vi "testSavedWithIdleTimeoutVisible.vi"(8 "error in (no error)":errorcluster, 11 "testStateMachineUtilities in":refnum<class "testStateMachineUtilities.lvclass">) -> (0 "error out":errorcluster, 3 "testStateMachineUtilities out":refnum<class "testStateMachineUtilities.lvclass">)   [LabVIEW 2013, in "testStateMachineUtilities.lvclass"]
uses:
  testStateMachineUtilities.lvclass
  <vilib>/Utility/traverseref.llb/TRef TravTarget.ctl
  <vilib>/Utility/traverseref.llb/VI Scripting - Traverse.lvlib
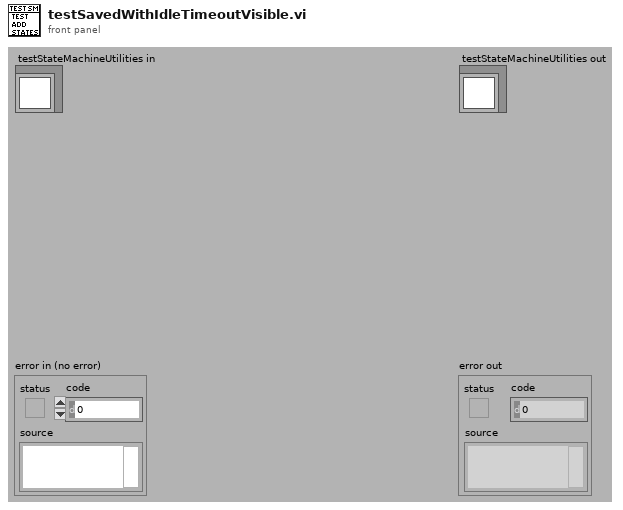
[diagram p1: front panel]
types:
  T1 = enum32{"Invalid", "Standard", "Closed", "Hidden", "Minimized", "Maximized"}
  T2 = typedef "TRef TravTarget.ctl" = enum16{"FP", "BD", "Other"}
  T3 = cluster{i32, refnum<vi>, "FrameNames":string[]}[]
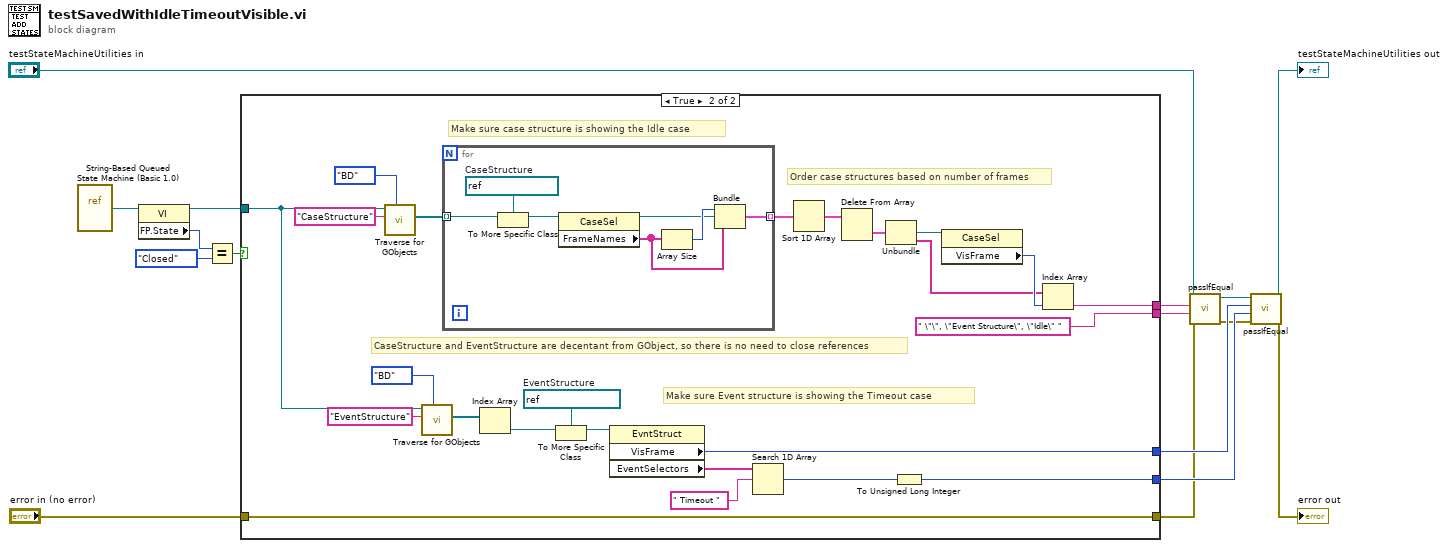
[diagram p0: block diagram]
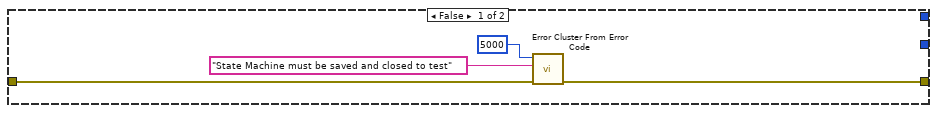
[diagram p2: hidden frame]
diagram:
  n1 = vi-ref "String-Based Queued State Machine (Basic 1.0).vi"() -> (w7:refnum<vi>)
  n2 = property class="VI"(reference=w7) -> (reference out=w4:refnum<vi>, "FP.State"=w6:T1)  [unwired: 1 in, 1 out]
  n3 = Equal?(x=w6, y=T1."Closed" ("Front Panel Window:State")) -> (x = y?=w3:bool)
  n4 = case shown="True" w3 {
    tunnel: [_ w27] -> w15
    tunnel: [_ " \"\", \"Event Structure\", \"Idle\" " ("y")] -> w14
    tunnel: [_ w25] -> w12
    tunnel: [_ w23] -> w11
    tunnel: w4 -> [_ w22]
    tunnel: [w19 w21] -> w2
    tunnel: "error in (no error)" -> [w20 w21]
    frame False {
      n5 = call <vilib>:"Error Cluster From Error Code.vi"("error in (no error)"=w20, "error message (\"\")"="State Machine must be saved and closed to test" ("error message (\"\")"), "error code (0)"=5000) -> ("error out"=w19:errorcluster)  [unwired: 6 in]
    }
    frame True {
      w32 = refnum<vi> refnum  # EventStructure
      # "Make sure Event structure is showing the Timeout case"
      # "Make sure case structure is showing the Idle case"
      # "Order case structures based on number of frames"
      # "CaseStructure and EventStructure are decentant from GObject, so there is no need to close references"
      n6 = call <vilib>:"Traverse for GObjects.vi"("Traverse Target"=TRef_TravTarget."BD", "Class Name"="CaseStructure", "VI Refnum"=w22) -> ("References"=w42:refnum<vi>[])  [unwired: 5 in, 3 out]
      n7 = call <vilib>:"Traverse for GObjects.vi"("Traverse Target"=TRef_TravTarget."BD", "Class Name"="EventStructure", "VI Refnum"=w22) -> ("References"=w31:refnum<vi>[])  [unwired: 5 in, 3 out]
      n8 = for {
        tunnel: w42 -> [w51] mode=indexing
        tunnel: [w47] -> w41 mode=indexing
        w50 = refnum<vi> refnum  # CaseStructure
        n9 = To More Specific Class(target class=w50, reference=w51) -> (specific class reference=w48:refnum<vi>)  [unwired: 1 in, 1 out]
        n10 = property class="CaseSel"(reference=w48) -> (reference out=w46:refnum<vi>, "FrameNames"=w45:string[])  [unwired: 1 in, 1 out]
        n11 = Array Size(array=w45) -> (size(s)=w49:i32)
        n12 = Bundle(w49, w46, "FrameNames"=w45) -> (w47:cluster{i32, refnum<vi>, "FrameNames":string[]})  [unwired: 1 in]
      }
      n13 = Index Array(array=w31) -> (element=w30:refnum<vi>)  [unwired: 1 in]
      n14 = To More Specific Class(target class=w32, reference=w30) -> (specific class reference=w33:refnum<vi>)  [unwired: 1 in, 1 out]
      n15 = property class="EvntStruct"(reference=w33) -> ("VisFrame"=w25:u32, "EventSelectors"=w29:string[])  [unwired: 1 in, 2 out]
      n16 = Search 1D Array(1D array=w29, element=" Timeout ") -> (index of element=w24:i32)  [unwired: 1 in]
      n17 = Sort 1D Array(array=w41) -> (sorted array=w40:T3)
      n18 = Delete From Array(array=w40) -> (deleted portion=w39:cluster{i32, refnum<vi>, "FrameNames":string[]})  [unwired: 2 in, 1 out]
      n19 = Unbundle(w39) -> (w38:refnum<vi>, "FrameNames"=w36:string[])  [unwired: 1 out]
      n20 = To Unsigned Long Integer(number=w24) -> (unsigned 32bit integer=w23:u32)
      n21 = property class="CaseSel"(reference=w38) -> ("VisFrame"=w37:u32)  [unwired: 1 in, 2 out]
      n22 = Index Array(array=w36, index=w37) -> (element=w27:string)
    }
  }
  n23 = call-dynamic "passIfEqual.vi"("error in (no error)"=w2, "y"=w14, "x"=w15, "TestCase in"="testStateMachineUtilities in") -> ("error out"=w10:errorcluster, "TestCase out"=w13:refnum<class "testStateMachineUtilities.lvclass">)  [unwired: 6 in]
  n24 = call-dynamic "passIfEqual.vi"("error in (no error)"=w10, "y"=w11, "x"=w12, "TestCase in"=w13) -> ("error out"=→"error out":errorcluster, "TestCase out"=→"testStateMachineUtilities out":refnum<class "testStateMachineUtilities.lvclass">)  [unwired: 6 in]
